vi "Test DB_CONNECTOR API.vi"() -> ()   [LabVIEW 2022 SP3, in "hse-db.lvlib"]
doc: "DB_CONNECTOR API Tester.\n\n____\nHAMPEL SOFTWARE ENGINEERING v1.4.0 (2023-12-19 09:52)"
uses:
  hse-db.lvlib
  <vilib>/Utility/error.llb/DialogType.ctl
  <vilib>/Hampel Software Engineering/HSE Logger/LogRecord/LogRecord.lvclass/LogRecord.ctl
  DB-Interface/DB-Interface.lvclass
  Query Poly-VIs/Query - String - 2D.vi
  DB_CONNECTOR.lvlib
  hse-libraries/Source/hse-dqmh/hse-dqmh.lvlib
  <vilib>/Hampel Software Engineering/HSE Logger/LogRecord/LogRecord.lvclass
  <vilib>/Hampel Software Engineering/HSE Logger/hse-logger.lvlib
panel:
  in  "Start and Configure":bool caption="btn_Query"
  in  "Show Main VI Diagram on Init (F)":bool
  in  "Rollback Transaction":bool
  in  "Module Timeout":i32
  in  "Set Module Timeout":bool
  in  "btn_Configure":bool caption="btn_Query"
  out "DB-Type":string
  in  "Get DB-Type":bool
  in  "btn_Fast_Query":bool caption="btn_Query"
  out "Query Time (ms)":u32
  out "Field Names":string[](array[string])
  in  "Config Section":string
  out "Meta Data":variant
  in  "btn_Commit_Transaction":bool caption="btn_Query"
  in  "btn_Start_Transaction":bool caption="btn_Query"
  out "Return Data":string[][](array[string])
  in  "btn_Query":bool
  in  "SQL Query":string
  in  "Run as Singleton?":bool
  in  "Show Block Diagram":bool
  in  "Refresh Modules":bool
  out "Active Modules":string[](array[string])
  in  "Stop Module":bool
  in  "Select Module":i32(ring)=-1 caption="Select Module\nTo send Request to" items=["All"=-1]
  in  "Run New Module":bool
  in  "Hide Module Panel":bool
  in  "Show Module Panel":bool
  out "Status":string
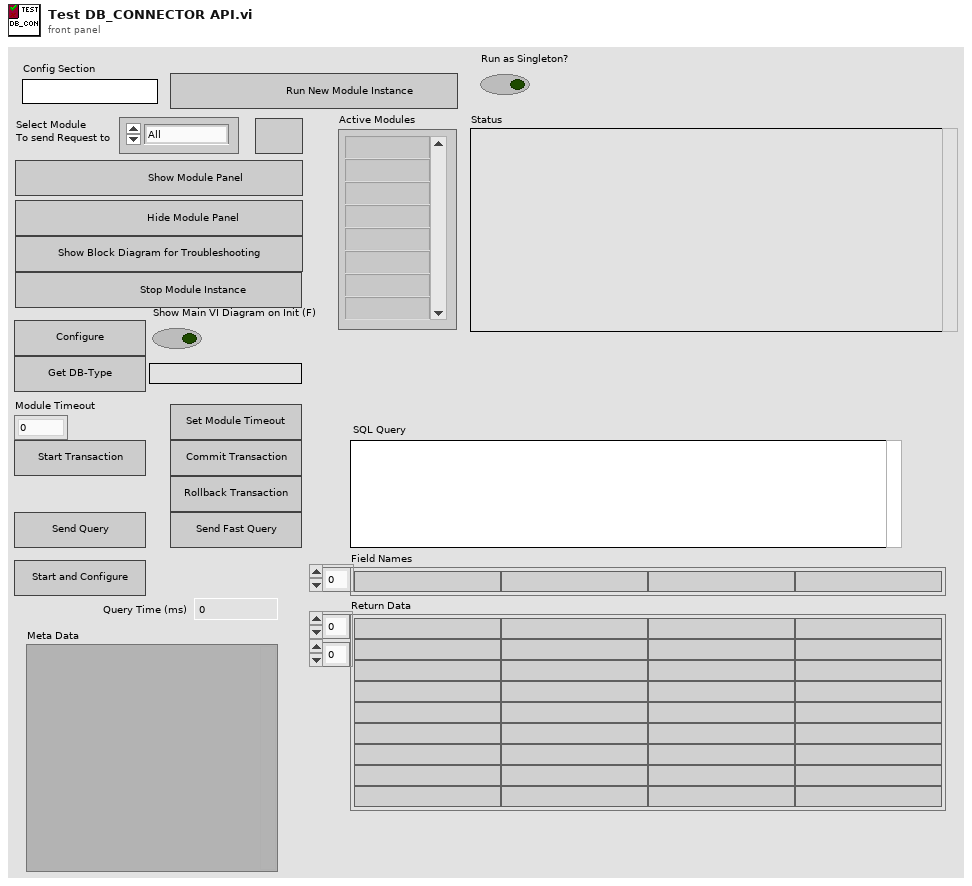
[diagram p1: front panel]
types:
  T1 = typedef "hse-db.lvlib/DB_CONNECTOR.lvlib/Broadcast Events--cluster.ctl" = cluster{"Module Did Init":refnum<user-event>, "Status Updated":refnum<user-event>, "Error Reported":refnum<user-event>, "Module Did Stop":refnum<user-event>, "Update Module Execution Status":refnum<user-event>, "Fast Query Reply":refnum<user-event>, "Configured and Connected":refnum<user-event>}
  T2 = typedef "DialogType.ctl" = u16
  T3 = typedef "hse-logger.lvlib/LogLevel.ctl" = enum16{"DEBUG", "INFO", "WARNING", "ERROR", "CRITICAL"}
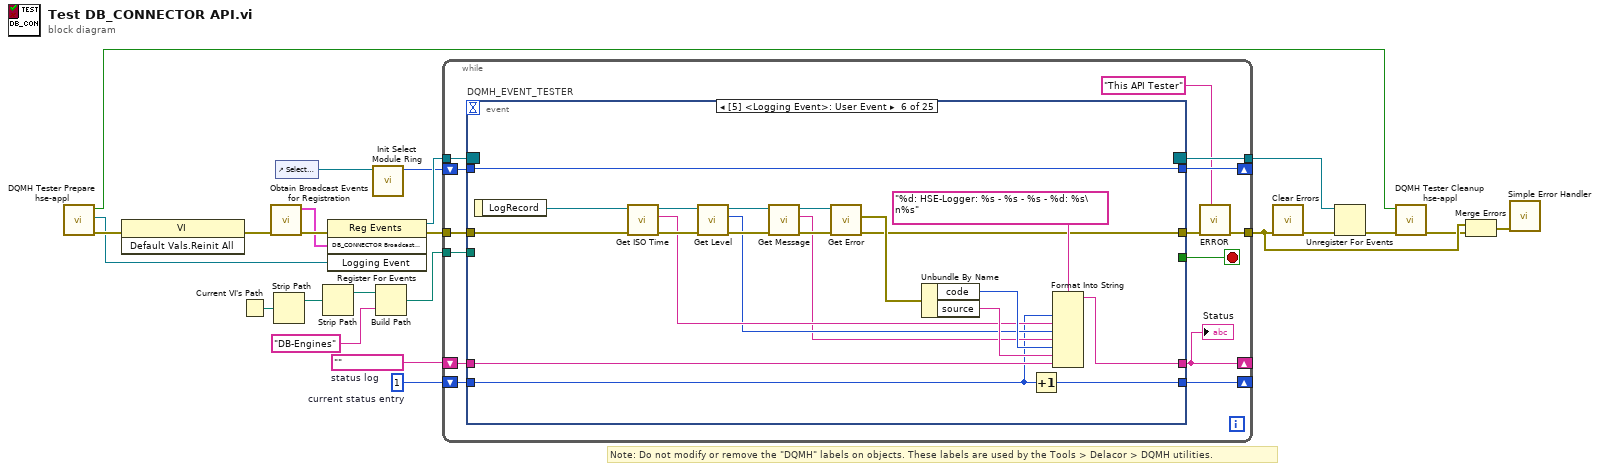
[diagram p0: block diagram]
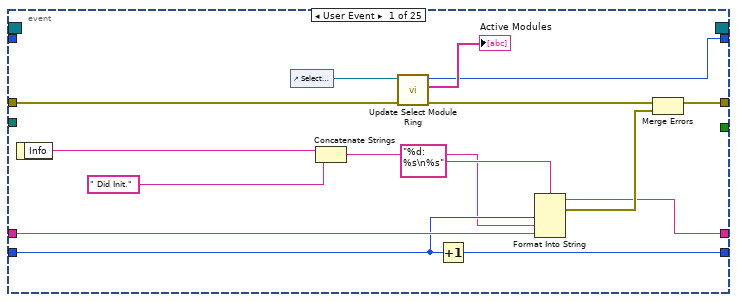
[diagram p2: hidden frame]
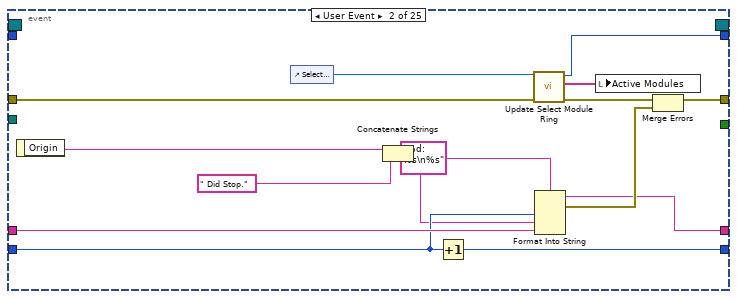
[diagram p3: hidden frame]
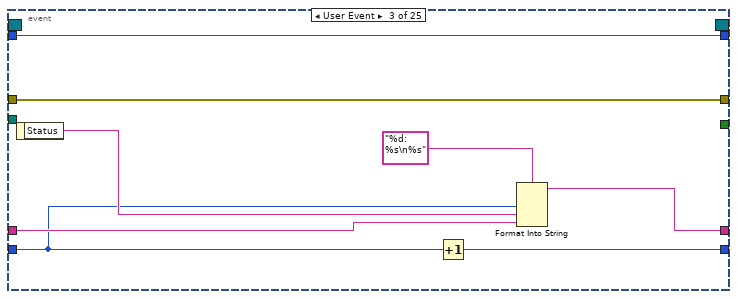
[diagram p4: hidden frame]
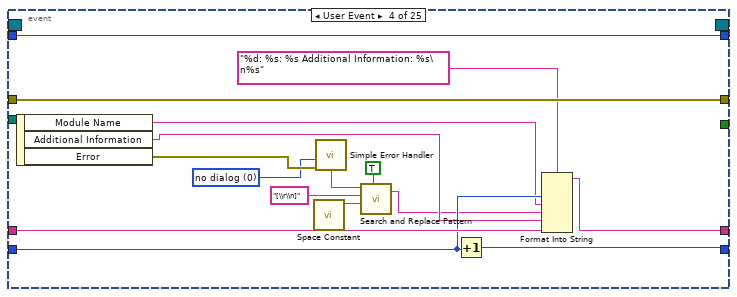
[diagram p5: hidden frame]
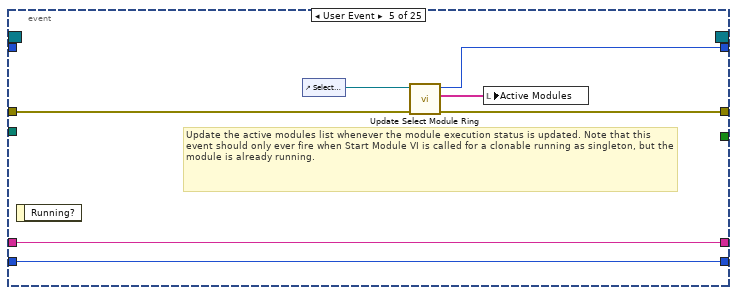
[diagram p6: hidden frame]
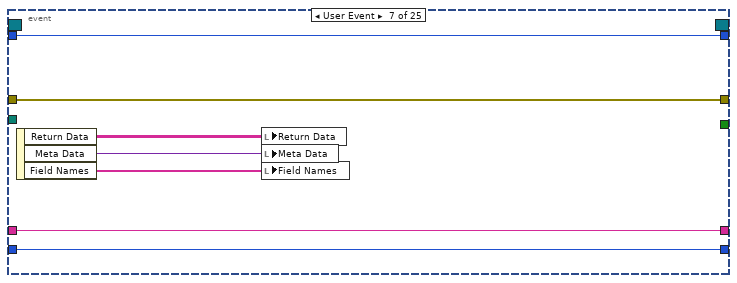
[diagram p7: hidden frame]
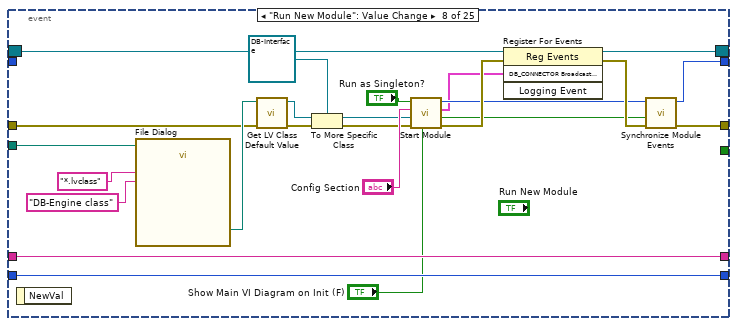
[diagram p8: hidden frame]
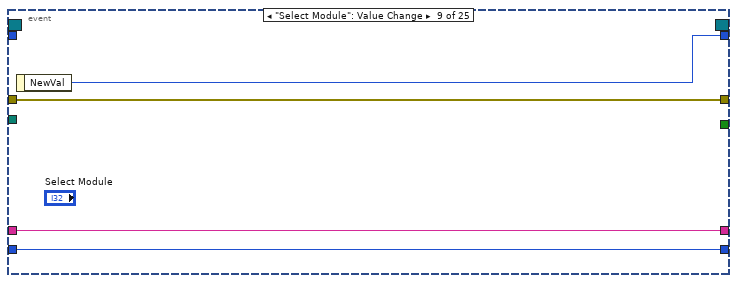
[diagram p9: hidden frame]
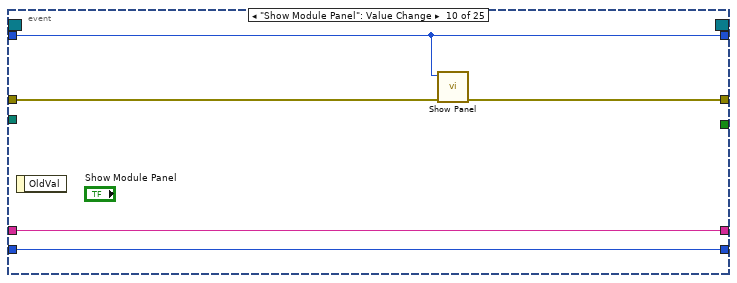
[diagram p10: hidden frame]
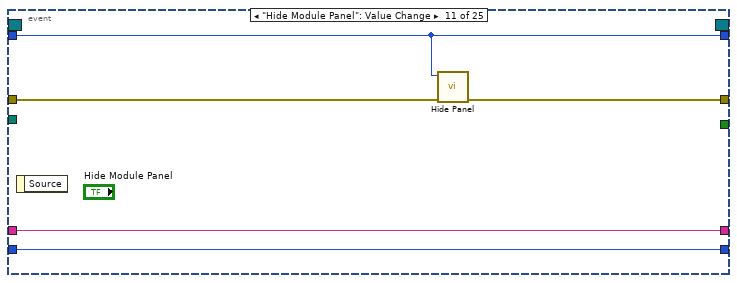
[diagram p11: hidden frame]
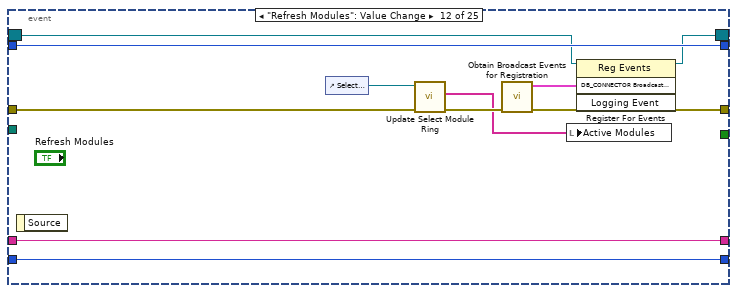
[diagram p12: hidden frame]
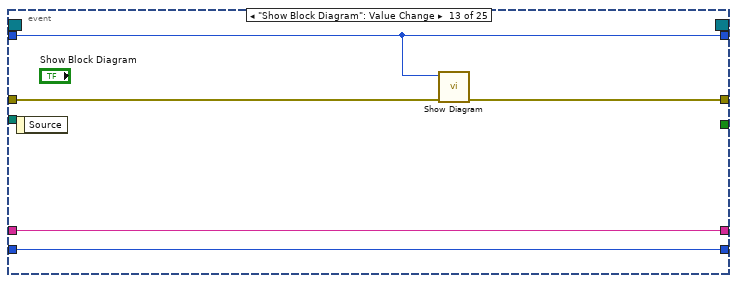
[diagram p13: hidden frame]
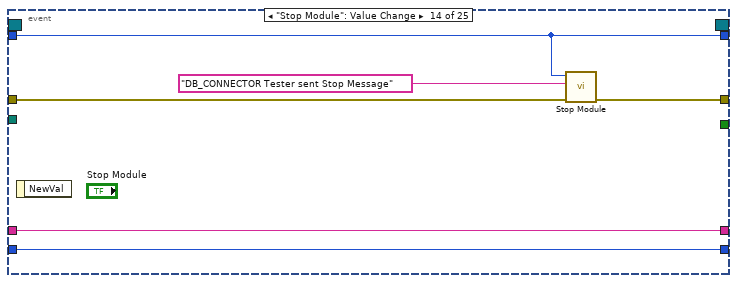
[diagram p14: hidden frame]
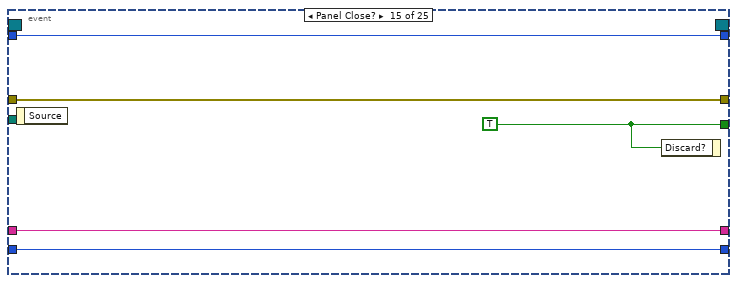
[diagram p15: hidden frame]
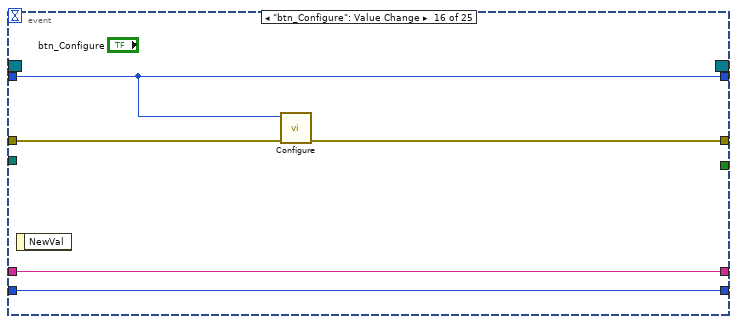
[diagram p16: hidden frame]
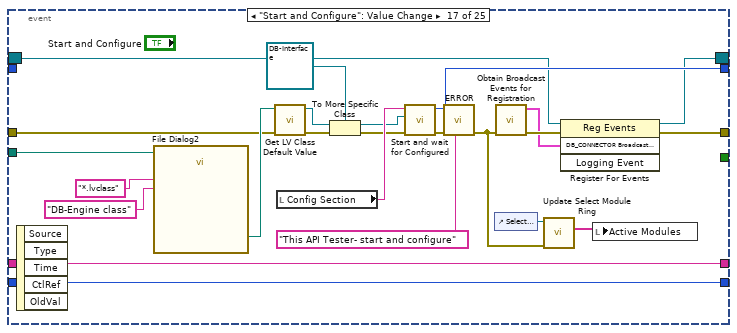
[diagram p17: hidden frame]
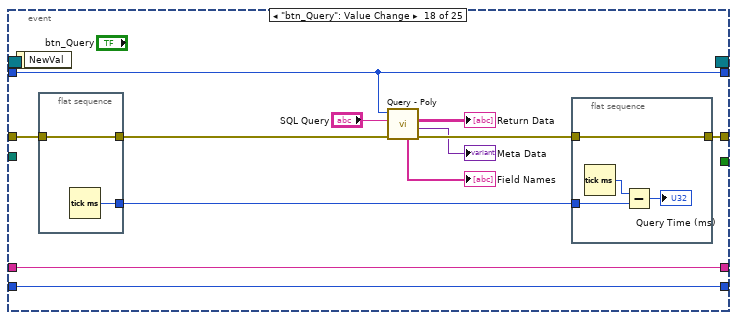
[diagram p18: hidden frame]
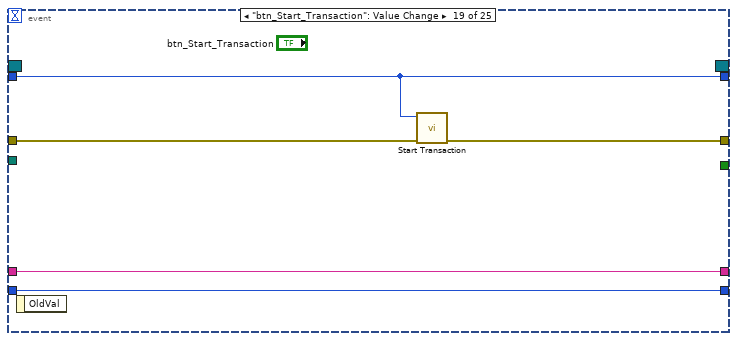
[diagram p19: hidden frame]
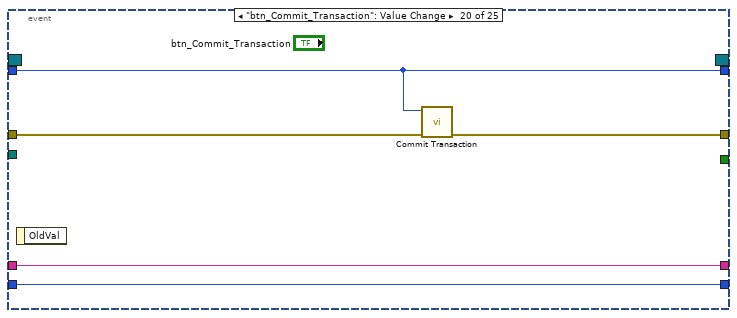
[diagram p20: hidden frame]
diagram:
  w20 = 1  # current status entry
  w21 = ""  # status log
  # "Note: Do not modify or remove the \"DQMH\" labels on objects. These labels are used by the Tools > Delacor > DQMH utilities."
  n1 = call "DQMH Tester Prepare hse-appl.vi"() -> ("error out"=w11:errorcluster, "Logging Event"=w2:refnum<user-event>, "Started?"=w8:bool)  [unwired: 8 in, 1 out]
  n2 = invoke class="VI" method="Default Vals.Reinit All"(error in=w11) -> (error out=w14:errorcluster)  [unwired: 2 in, 2 out]
  n3 = Current VI's Path() -> (path=w6:path)
  n4 = call "Obtain Broadcast Events for Registration.vi"("error in (no error)"=w14) -> ("error out"=w13:errorcluster, "DB_CONNECTOR Broadcast Events"=w1:T1)  [unwired: 9 in]
  n5 = Strip Path(path=w6) -> (stripped path=w7:path)  [unwired: 1 out]
  n6 = control-ref of="Select Module"() -> (w18:refnum<vi>)
  n7 = Strip Path(path=w7) -> (stripped path=w5:path)  [unwired: 1 out]
  n8 = register-events(error in=w13, w1, w2) -> (reference out=w23:refnum<event-registration>, error out=w17:errorcluster)  [unwired: 1 in]
  n9 = call "Init Select Module Ring.vi"("Select Module Ring Ref"=w18) -> ("Value for All Modules"=w19:i32)  [unwired: 8 in, 2 out]
  n10 = Build Path(base path=w5, name or relative path="DB-Engines" ("pattern (all files)")) -> (appended path=w3:path)
  n11 = while {
    tunnel: w23 -> [w37]
    tunnel: [w26] -> w15
    tunnel: w17 -> [w36]
    shift-right: [w32] -> _
    shift-left: w21 -> [w34]
    shift-right: [w33] -> _
    shift-left: w20 -> [w35]
    shift-right: [w30] -> _
    shift-left: w19 -> [w31]
    tunnel: [w29] -> w16
    tunnel: w3 -> [w27]
    stop <- w24 stop-if-true
    n12 = event "DQMH_EVENT_TESTER" shown="[5] <Logging Event>: User Event" {
      selector: w37 -> [_ _ _ _ _ _ _ w146 _ _ _ w170 _ _ _ _ w202 _ _ _ _ _ _ _ _]
      dyn-events: [_ _ _ _ _ _ _ w145 _ _ _ w169 _ _ _ _ w203 _ _ _ _ _ _ _ _] -> w29
      timeout: _ -> [_ _ _ _ _ _ _ _ _ _ _ _ _ _ _ _ _ _ _ _ _ _ _ _ _]
      tunnel: [_ _ _ _ _ _ _ _ _ _ _ _ _ _ w191 _ _ _ _ _ _ _ _ _ _] -> w24
      tunnel: [w41 w59 w75 w90 w94 w101 w126 w138 w154 w158 w163 w166 w177 w182 w190 w193 w205 w221 w239 w243 w249 w265 w271 w276 w288] -> w28
      tunnel: w36 -> [w43 w61 w75 w90 w95 w99 w126 w130 w154 w159 w164 w171 w180 w183 w190 w194 w208 w223 w242 w244 w252 w268 w274 w279 w288]
      tunnel: w35 -> [w49 w64 w68 w87 w97 w104 w124 w147 w152 w156 w161 w174 w178 w185 w188 w195 w218 w229 w240 w246 w255 w266 w272 w277 w285]
      tunnel: w34 -> [w50 w65 w71 w89 w98 w105 w125 w148 w153 w157 w162 w175 w179 w186 w189 w196 w219 w230 w241 w247 w256 w267 w273 w278 w287]
      tunnel: [w47 w62 w72 w88 w98 w102 w125 w148 w153 w157 w162 w175 w179 w186 w189 w196 w219 w230 w241 w247 w256 w267 w273 w278 w286] -> w32
      tunnel: [w48 w63 w74 w86 w97 w103 w124 w147 w152 w156 w161 w174 w178 w185 w188 w195 w218 w229 w240 w246 w255 w266 w272 w277 w284] -> w33
      tunnel: w31 -> [_ _ w69 w91 _ w119 w123 _ _ w155 w160 w173 w176 w184 w187 w192 _ w228 w238 w245 w254 w264 w270 w275 w280]
      tunnel: [w38 w56 w69 w91 w93 w119 w123 w140 w151 w155 w160 w173 w176 w184 w187 w192 w207 w228 w238 w245 w254 w264 w270 w275 w280] -> w30
      tunnel: w27 -> [_ _ _ _ _ _ _ w131 _ _ _ _ _ _ _ _ w211 _ _ _ _ _ _ _ _]
      event User Event {
        n13 = event-data() -> ("Info"=w46:string)  [unwired: 1 in]
        n14 = control-ref of="Select Module"() -> (w40:refnum<vi>)
        n15 = Concatenate Strings(w46, " Did Init.") -> (w45:string)
        n16 = call "Update Select Module Ring.vi"("error in (no error)"=w43, "Select Module Ring Ref"=w40) -> ("error out"=w42:errorcluster, "Active Modules (Array)"=→"Active Modules":string[], "New Module Ring Value"=w38:i32)  [unwired: 7 in]
        n17 = Increment(x=w49) -> (x+1=w48:i32)
        n18 = Format Into String(format string="%d: %s\n%s", w49, w45, w50) -> (resulting string=w47:string, error out=w52:errorcluster)  [unwired: 2 in]
        n19 = Merge Errors(w42, w52) -> (w41:errorcluster)
      }
      event User Event {
        n20 = event-data() -> ("Origin"=w54:string)  [unwired: 1 in]
        n21 = control-ref of="Select Module"() -> (w58:refnum<vi>)
        n22 = Concatenate Strings(w54, " Did Stop.") -> (w53:string)
        n23 = Increment(x=w64) -> (x+1=w63:i32)
        n24 = call "Update Select Module Ring.vi"("error in (no error)"=w61, "Select Module Ring Ref"=w58) -> ("error out"=w60:errorcluster, "Active Modules (Array)"=w57:string[], "New Module Ring Value"=w56:i32)  [unwired: 7 in]
        n25 = Format Into String(format string="%d: %s\n%s", w64, w53, w65) -> (resulting string=w62:string, error out=w67:errorcluster)  [unwired: 2 in]
        n26 = local write "Active Modules"(w57) -> ()
        n27 = Merge Errors(w60, w67) -> (w59:errorcluster)
      }
      event User Event {
        n28 = event-data() -> ("Status"=w70:string)  [unwired: 1 in]
        n29 = Increment(x=w68) -> (x+1=w74:i32)
        n30 = Format Into String(format string="%d: %s\n%s", w68, w70, w71) -> (resulting string=w72:string)  [unwired: 2 in, 1 out]
      }
      event User Event {
        w82 = T2 0 items=["no dialog", "OK message", "continue or stop message", "OK message + warnings", "continue/stop + warnings"] ("type of dialog (OK msg:1)")
        n31 = event-data() -> ("Module Name"=w83:string, "Additional Information"=w84:string, "Error"=w85:errorcluster)  [unwired: 1 in]
        n32 = call <vilib>:"Space Constant.vi"() -> ("String"=w78:string)
        n33 = call <vilib>:"Simple Error Handler.vi"("type of dialog (OK msg:1)"=w82, "error in (no error)"=w85) -> ("message"=w81:string)  [unwired: 3 in, 4 out]
        n34 = call <vilib>:"Search and Replace Pattern.vi"("string"=w81, "regular expression (\"\")"="[\\r\\n]" ("regular expression (\"\")"), "replace string (\"\")"=w78, "replace all? (F)"=TRUE ("replace all CR/LF with spaces")) -> ("result string"=w80:string)  [unwired: 1 in, 1 out]
        n35 = Increment(x=w87) -> (x+1=w86:i32)
        n36 = Format Into String(format string="%d: %s: %s Additional Information: %s\n%s", w87, w83, w80, w84, w89) -> (resulting string=w88:string)  [unwired: 2 in, 1 out]
      }
      event User Event {
        # "Update the active modules list whenever the module execution status is updated. Note that this event should only ever fire when Start Module VI is called for a clonable running as singleton, but the module is already running."
        n37 = event-data() -> ()  [unwired: 1 in, 1 out]
        n38 = control-ref of="Select Module"() -> (w96:refnum<vi>)
        n39 = call "Update Select Module Ring.vi"("error in (no error)"=w95, "Select Module Ring Ref"=w96) -> ("error out"=w94:errorcluster, "Active Modules (Array)"=w92:string[], "New Module Ring Value"=w93:i32)  [unwired: 7 in]
        n40 = local write "Active Modules"(w92) -> ()
      }
      event User Event {
        n41 = event-data() -> ("LogRecord"=w100:refnum<class "LogRecord.lvclass">)  [unwired: 1 in]
        n42 = call <vilib>:"Get ISO Time.vi"("error in"=w99, "LogRecord in"=w100) -> ("error out"=w118:errorcluster, "ISO Time"=w108:string, "LogRecord out"=w117:refnum<class "LogRecord.lvclass">)  [unwired: 7 in]
        n43 = call <vilib>:"Get Level.vi"("error in"=w118, "LogRecord in"=w117) -> ("error out"=w115:errorcluster, "Level"=w107:T3, "LogRecord out"=w116:refnum<class "LogRecord.lvclass">)  [unwired: 7 in]
        n44 = call <vilib>:"Get Message.vi"("error in"=w115, "LogRecord in"=w116) -> ("error out"=w113:errorcluster, "Message"=w106:string, "LogRecord out"=w114:refnum<class "LogRecord.lvclass">)  [unwired: 7 in]
        n45 = call <vilib>:"Get Error.vi"("error in"=w113, "LogRecord in"=w114) -> ("error out"=w101:errorcluster, "Error"=w109:errorcluster)  [unwired: 7 in, 1 out]
        n46 = Unbundle By Name(w109) -> ("code"=w111:i32, "source"=w110:string)
        n47 = Increment(x=w104) -> (x+1=w103:i32)
        n48 = Format Into String(format string="%d: HSE-Logger: %s - %s - %s - %d: %s\n%s", w104, w108, w107, w106, w111, w110, w105) -> (resulting string=w102:string)  [unwired: 2 in, 1 out]
      }
      event User Event {
        n49 = event-data() -> ("Return Data"=w122:string[][], "Meta Data"=w121:variant, "Field Names"=w120:string[])  [unwired: 1 in]
        n50 = local write "Return Data"(w122) -> ()
        n51 = local write "Meta Data"(w121) -> ()
        n52 = local write "Field Names"(w120) -> ()
      }
      event "Run New Module": Value Change {
        n53 = event-data() -> ()  [unwired: 1 in, 1 out]
        n54 = call "File Dialog"("start path"=w131, "pattern (all files)"="*.lvclass", "pattern label"="DB-Engine class") -> ("selected path"=w134:path)  [unwired: 9 in, 3 out]
        n55 = call <vilib>:"Get LV Class Default Value.vi"("error in (no error)"=w130, "class path"=w134) -> ("error out"=w129:errorcluster, "object"=w137:refnum<class>)  [unwired: 8 in]
        n56 = To More Specific Class(target class=refnum<class "DB-Interface.lvclass"> refnum ("DB-Engine"), reference=w137, error in=w129) -> (specific class reference=w135:refnum<class "DB-Interface.lvclass">, error out=w128:errorcluster)
        n57 = call "Start Module.vi"("Show Main VI Diagram on Init (F)"="Show Main VI Diagram on Init (F)", "error in (no error)"=w128, "DB-Engine"=w135, "Config Section"="Config Section", "Run as Singleton? (F)"="Run as Singleton?") -> ("error out"=w149:errorcluster, "Wait for Event Sync?"=w143:bool, "DB_CONNECTOR Broadcast Events"=w142:T1, "Module ID"=w144:i32)  [unwired: 3 in]
        n58 = register-events(reference=w146, error in=w149, w142) -> (reference out=w145:refnum<event-registration>, error out=w150:errorcluster)  [unwired: 1 in]
        n59 = call "Synchronize Module Events.vi"("error in (no error)"=w150, "Wait for Event Sync?"=w143, "Module ID"=w144) -> ("error out"=w138:errorcluster, "Module ID (dup)"=w140:i32)  [unwired: 7 in]
      }
      event "Select Module": Value Change {
        n60 = event-data() -> ("NewVal"=w151:i32)  [unwired: 1 in]
      }
      event "Show Module Panel": Value Change {
        n61 = event-data() -> ()  [unwired: 1 in, 1 out]
        n62 = call "Show Panel.vi"("error in (no error)"=w159, "Module ID"=w155) -> ("error out"=w158:errorcluster)  [unwired: 9 in]
      }
      event "Hide Module Panel": Value Change {
        n63 = event-data() -> ()  [unwired: 1 in, 1 out]
        n64 = call "Hide Panel.vi"("error in (no error)"=w164, "Module ID"=w160) -> ("error out"=w163:errorcluster)  [unwired: 9 in]
      }
      event "Refresh Modules": Value Change {
        n65 = event-data() -> ()  [unwired: 1 in, 1 out]
        n66 = control-ref of="Select Module"() -> (w172:refnum<vi>)
        n67 = call "Update Select Module Ring.vi"("error in (no error)"=w171, "Select Module Ring Ref"=w172) -> ("error out"=w167:errorcluster, "Active Modules (Array)"=w165:string[])  [unwired: 7 in, 1 out]
        n68 = call "Obtain Broadcast Events for Registration.vi"("error in (no error)"=w167) -> ("error out"=w166:errorcluster, "DB_CONNECTOR Broadcast Events"=w168:T1)  [unwired: 9 in]
        n69 = local write "Active Modules"(w165) -> ()
        n70 = register-events(reference=w170, w168) -> (reference out=w169:refnum<event-registration>)  [unwired: 2 in, 1 out]
      }
      event "Show Block Diagram": Value Change {
        n71 = event-data() -> ()  [unwired: 1 in, 1 out]
        n72 = call "Show Diagram.vi"("error in (no error)"=w180, "Module ID"=w176) -> ("error out"=w177:errorcluster)  [unwired: 9 in]
      }
      event "Stop Module": Value Change {
        n73 = event-data() -> ()  [unwired: 1 in, 1 out]
        n74 = call "Stop Module.vi"("error in (no error)"=w183, "Origin"="DB_CONNECTOR Tester sent Stop Message", "Module ID"=w184) -> ("error out"=w182:errorcluster)  [unwired: 8 in]
      }
      event Panel Close? {
        w191 = TRUE ("Discard?")
        n75 = event-data() -> ()  [unwired: 1 in, 1 out]
        n76 = event-data("Discard?"=w191) -> ()  [unwired: 1 in, 1 out]
      }
      event "btn_Configure": Value Change {
        n77 = event-data() -> ()  [unwired: 1 in, 1 out]
        n78 = call "Configure.vi"("error in (no error)"=w194, "Module ID"=w192) -> ("error out"=w193:errorcluster)  [unwired: 8 in, 1 out]
      }
      event "Start and Configure": Value Change {
        n79 = event-data() -> ()  [unwired: 1 in, 5 out]
        n80 = call "File Dialog2"("start path"=w211, "pattern (all files)"="*.lvclass", "pattern label"="DB-Engine class") -> ("selected path"=w215:path)  [unwired: 9 in, 3 out]
        n81 = call <vilib>:"Get LV Class Default Value.vi"("class path"=w215) -> ("error out"=w212:errorcluster, "object"=w217:refnum<class>)  [unwired: 9 in]
        n82 = local read "Config Section"() -> (w210:string)
        n83 = To More Specific Class(target class=refnum<class "DB-Interface.lvclass"> refnum ("DB-Engine"), reference=w217, error in=w212) -> (specific class reference=w209:refnum<class "DB-Interface.lvclass">)  [unwired: 1 out]
        n84 = call "Start and wait for Configured.vi"("error in"=w208, "DB-Engine"=w209, "Config Section"=w210) -> ("error out"=w199:errorcluster, "Module ID"=w207:i32)  [unwired: 7 in]
        n85 = call <vilib>:"ERROR.vi"("Message"="This API Tester- start and configure", "error in"=w199) -> ("error out"=w198:errorcluster)  [unwired: 9 in]
        n86 = control-ref of="Select Module"() -> (w200:refnum<vi>)
        n87 = call "Obtain Broadcast Events for Registration.vi"("error in (no error)"=w198) -> ("error out"=w206:errorcluster, "DB_CONNECTOR Broadcast Events"=w204:T1)  [unwired: 9 in]
        n88 = call "Update Select Module Ring.vi"("error in (no error)"=w198, "Select Module Ring Ref"=w200) -> ("Active Modules (Array)"=w201:string[])  [unwired: 7 in, 2 out]
        n89 = register-events(reference=w202, error in=w206, w204) -> (reference out=w203:refnum<event-registration>, error out=w205:errorcluster)  [unwired: 1 in]
        n90 = local write "Active Modules"(w201) -> ()
      }
      event "btn_Query": Value Change {
        n91 = event-data() -> ()  [unwired: 1 in, 1 out]
        n92 = flat-sequence {
          tunnel: w223 -> [w237]
          tunnel: [w237] -> w222
          tunnel: [w236] -> w220
          frame #0 {
            n93 = Tick Count (ms)() -> (millisecond timer value=w236:u32)
          }
        }
        n94 = call-poly "Query - Poly.vi"("error in"=w222, "Query"="SQL Query", "Module ID"=w228) -> ("error out"=w231:errorcluster, "Meta Data"=→"Meta Data":variant, "Return Data"=→"Return Data":string[][], "Field Names"=→"Field Names":string[])  [unwired: 5 in]
        n95 = flat-sequence {
          tunnel: w231 -> [w235]
          tunnel: [w235] -> w221
          tunnel: w220 -> [w233]
          frame #0 {
            n96 = Tick Count (ms)() -> (millisecond timer value=w234:u32)
            n97 = Subtract(x=w234, y=w233) -> (x-y=→"Query Time (ms)":u32)
          }
        }
      }
      event "btn_Start_Transaction": Value Change {
        n98 = event-data() -> ()  [unwired: 1 in, 1 out]
        n99 = call "Start Transaction.vi"("error in (no error)"=w242, "Module ID"=w238) -> ("error out"=w239:errorcluster)  [unwired: 9 in]
      }
      event "btn_Commit_Transaction": Value Change {
        n100 = event-data() -> ()  [unwired: 1 in, 1 out]
        n101 = call "Commit Transaction.vi"("error in (no error)"=w244, "Module ID"=w245) -> ("error out"=w243:errorcluster)  [unwired: 7 in, 2 out]
      }
      event "btn_Fast_Query": Value Change {
        n102 = event-data() -> ()  [unwired: 1 in, 1 out]
        n103 = flat-sequence {
          tunnel: w252 -> [w262]
          tunnel: [w262] -> w251
          tunnel: [w261] -> w248
          frame #0 {
            n104 = Tick Count (ms)() -> (millisecond timer value=w261:u32)
          }
        }
        n105 = local read "SQL Query"() -> (w253:string)
        n106 = call "Fast Query.vi"("error in (no error)"=w251, "Query"=w253, "Module ID"=w254) -> ("error out"=w250:errorcluster)  [unwired: 8 in]
        n107 = flat-sequence {
          tunnel: w250 -> [w260]
          tunnel: [w260] -> w249
          tunnel: w248 -> [w258]
          frame #0 {
            n108 = Tick Count (ms)() -> (millisecond timer value=w259:u32)
            n109 = Subtract(x=w259, y=w258) -> (x-y=w257:u32)
            n110 = local write "Query Time (ms)"(w257) -> ()
          }
        }
      }
      event "Get DB-Type": Value Change {
        n111 = event-data() -> ()  [unwired: 1 in, 1 out]
        n112 = call "Get DB-Type.vi"("error in (no error)"=w268, "Module ID"=w264) -> ("error out"=w265:errorcluster, "DB-Type"=→"DB-Type":string)  [unwired: 8 in]
      }
      event "Set Module Timeout": Value Change {
        n113 = event-data() -> ()  [unwired: 1 in, 1 out]
        n114 = call "Set Module Timeout.vi"("error in (no error)"=w274, "Module Timeout"="Module Timeout", "Module ID"=w270) -> ("error out"=w271:errorcluster)  [unwired: 8 in]
      }
      event "Rollback Transaction": Value Change {
        n115 = event-data() -> ()  [unwired: 1 in, 1 out]
        n116 = call "Rollback Transaction.vi"("error in"=w279, "Module ID"=w275) -> ("error out"=w276:errorcluster)  [unwired: 8 in, 1 out]
      }
      event User Event {
        n117 = event-data() -> ()  [unwired: 1 in, 1 out]
        n118 = Format Into String(format string="module %d configured and connected", w280) -> (resulting string=w281:string)  [unwired: 2 in, 1 out]
        n119 = Increment(x=w285) -> (x+1=w284:i32)
        n120 = Format Into String(format string="%d: %s\n%s", w285, w281, w287) -> (resulting string=w286:string)  [unwired: 2 in, 1 out]
      }
    }
    "Status" <- w32
    n121 = call <vilib>:"ERROR.vi"("Message"="This API Tester" ("Origin"), "error in"=w28) -> ("error out"=w26:errorcluster)  [unwired: 9 in]
  }
  n122 = call <vilib>:"Clear Errors.vi"("error in (no error)"=w15) -> ("error out"=w22:errorcluster)  [unwired: 5 in, 1 out]
  n123 = Unregister For Events(event registration refnum=w16, error in=w22) -> (error out=w10:errorcluster)
  n124 = call "DQMH Tester Cleanup hse-appl.vi"("error in"=w10, "Stop?"=w8) -> ("error out"=w9:errorcluster)  [unwired: 9 in]
  n125 = Merge Errors(w15, w9) -> (w12:errorcluster)
  n126 = call <vilib>:"Simple Error Handler.vi"("error in (no error)"=w12) -> ()  [unwired: 4 in, 5 out]
